vi "subSave_AcquireMC3DZInfomation.vi"(3 "Z-Stack":T1={"Z end"=0.0, "Step Num"=1, "Step Size"=2.0, "Z0"=3471.0, "z-stack?"=FALSE}) -> (1 "Z info":string)   [LabVIEW 2015]
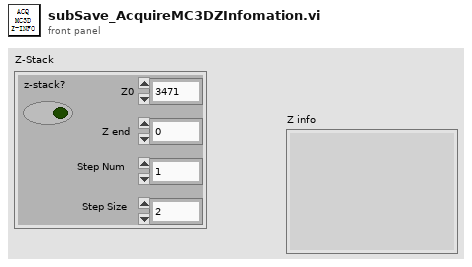
[diagram p1: front panel]
types:
  T1 = cluster{"Z end":dbl, "Step Num":i32, "Step Size":dbl, "Z0":dbl, "z-stack?":bool}
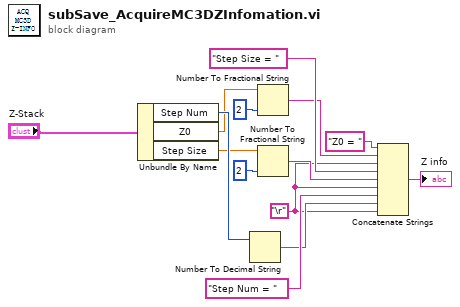
[diagram p0: block diagram]
diagram:
  w6 = "\r"
  n1 = Unbundle By Name("Z-Stack") -> ("Step Num"=w5:i32, "Z0"=w4:dbl, "Step Size"=w3:dbl)
  n2 = Number To Decimal String(number=w5) -> (decimal integer string=w13:string)  [unwired: 1 in]
  n3 = Number To Fractional String(number=w4, precision (6)=i16 2 ("width (-)")) -> (F-format string=w7:string)  [unwired: 2 in]
  n4 = Number To Fractional String(number=w3, precision (6)=i16 2 ("width (-)")) -> (F-format string=w12:string)  [unwired: 2 in]
  n5 = Concatenate Strings("Z0 = " ("string"), w7, w6, "Step Size = " ("string"), w12, w6, "Step Num = " ("string"), w13, w6) -> (→"Z info":string)
